vi "Read From Start to Stop.vi"(0 "RedPitaya TCP Connection in":refnum<k5>, 3 "Start Position":u16, 4 "Stop Position":u16, 5 "error in":errorcluster, 8 "Channel #":u16(ring)=1 items=["Channel 1"=1, "Channel 2"=2], 12 "timeout ms (2000)":i32=2000) -> (14 "RedPitaya TCP Connection out":refnum<k5>, 16 "Measurement Array":dbl[](array[numeric]), 19 "error out":errorcluster)   [LabVIEW 2021, in "RedPitaya.lvlib"]
doc: "Read samples from start to stop position in buffer."
uses:
  RedPitaya.lvlib
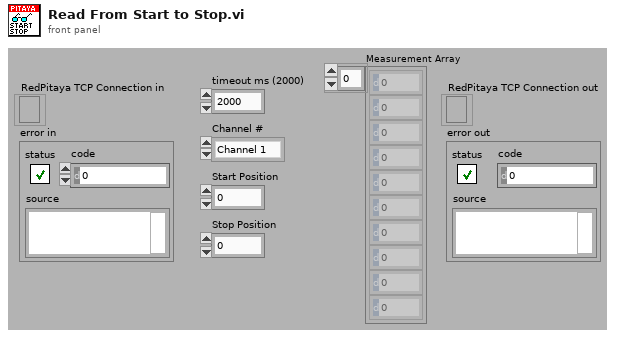
[diagram p1: front panel]
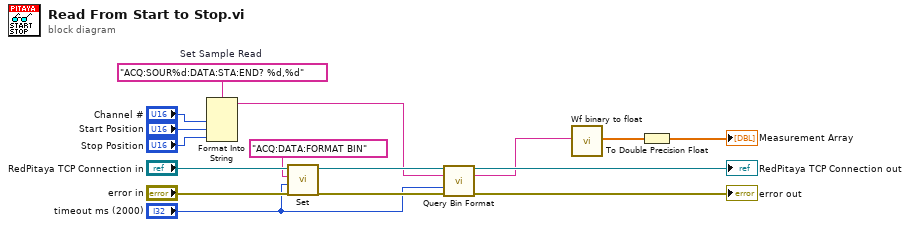
[diagram p0: block diagram]
diagram:
  w16 = "ACQ:SOUR%d:DATA:STA:END? %d,%d"  # Set Sample Read
  n1 = Format Into String(format string=w16, "Channel #", "Start Position", "Stop Position") -> (resulting string=w7:string)  [unwired: 2 in, 1 out]
  n2 = call "Set.vi"("error in"="error in", "timeout ms (2000)"="timeout ms (2000)", "SCPI Message"="ACQ:DATA:FORMAT BIN", "RedPitaya connection in"="RedPitaya TCP Connection in") -> ("error out"=w6:errorcluster, "RedPitaya connection out"=w9:refnum<k5>)  [unwired: 5 in, 1 out]
  n3 = call "Query Bin Format.vi"("RedPitaya connection in"=w9, "SCPI Query"=w7, "timeout ms (2000)"="timeout ms (2000)", "error in"=w6) -> ("RedPitaya connection out"=→"RedPitaya TCP Connection out":refnum<k5>, "data out"=w3:string, "error out"=→"error out":errorcluster)  [unwired: 9 in]
  n4 = call "Wf binary to float.vi"("Input string"=w3) -> ("Data out"=w2:sgl[])  [unwired: 18 in]
  n5 = To Double Precision Float(number=w2) -> (double precision float=→"Measurement Array":dbl[])
